vi "commander7.vi"() -> ()   [LabVIEW 2015]
uses:
  G_DATA.vi
  G_LCM.vi
  G_VEH.vi
  G_NAV.vi
  G_PATH.vi
  <vilib>/addons/control/pid/pid.llb/PID (DBL).vi
  G_SEN.vi
  <vilib>/addons/control/pid/NI_PID_pid.lvlib
panel:
  in  "handle":dbl
  in  "shifthold":dbl=0.02
  out "String":string="콜 서비스 대기 중"
  out "EURECAR_VISION":T1
  out "count":i32
  out "P2V Sign":picture[](array[picture])=[bytes[7530], bytes[7530], bytes[7530], bytes[7530]]
  out "Array 2":picture[](array[picture])
  out "sign 2":picture[](array[picture])
  out "sign":picture[](array[picture])
  in  "TTL":bool
  in  "Steering gain":dbl=0.8
  out "obs shift":dbl format="%.2f"
  in  "lane keep":bool
  in  "replay":bool
  in  "x":dbl min=-5.0 max=5.0 step=1.0
  out "display":u32=10
  out "control":u32=10
  out "update":bool=TRUE
  in  "save lcm":bool
  out "LCM Recv Data":string="GGA_2\t266\rSDT_GPS_DATA\t268\rGGA_1\t268\rRMC_2\t259\rRMC_1\t262\rEYE_RAW_T\t537\rPATH_T\t1344\rIBEO_2202_T\t672\rPOS_T\t3572\rCON_T\t4009\rCAN_T\t4707\r"
  out "GPS DATA 2":T2={"type"="WAAS", "x_lcc"=-395.2637182511565, "y_lcc"=-852.8277788987846, "latdev"=0.99, "londev"=0.99, "sats"=11, "gps_l1_ranges"=0, "gps_l1_mask_ranges"=0, "gps_l2_mask_ranges"=0, "Heading"=151.74409645131422, "lon"=127.35651, "lat"=36.36776, "time"="15:03:34.8", "hgps"=151.54, "lag"=0.0, "MAP"="KAIST"} {"lag" format="%#_5g"; "hgps" format="%#_5g"; "lat" format="%#_11g"; "lon" format="%#_11g"; "Heading" format="%#_5g"; "latdev" format="%#_4g"; "londev" format="%#_4g"}
  in  "Obs":bool=TRUE
  in  "Log":bool
  out "path":u32=10
  out "sensor":u32=10 format="%02.0f"
  out "Speed limit":dbl=20.0
  out "collision":bool
  in  "Load Path":bool
  in  "Max. Vel.":dbl=20.0 min=-5.0 max=120.0 step=5.0
  in  "RESET PATH":bool
  out "col":i16(graph)
  out "stop":bool
  in  "Reverse":bool
  in  "STOP":bool
  out "Waveform Chart 4":cluster{"auto":i16, "run":i16}(graph)={"auto"=1, "run"=0}
  out "Waveform Chart 3":cluster{"Steer_input":dbl, dbl, "handle":dbl}(graph)
  out "Waveform Chart 2":T3(graph)={"VS_des"=0.0, "VS_can"=31.498562500000002, "VS_des"=20.0}
  out "Heading":cluster{"Heading":dbl, "hgps":dbl}(graph)={"Heading"=151.74409645131422, "hgps"=151.54}
  out "XY Graph 2":cluster{"Y":dbl[], "Y":dbl[]}[](graph)=[{"Y"=[-395.3040396828474], "Y"=[-852.7527551292769]}, {"Y"=array[29298 elements], "Y"=array[29298 elements]}, {"Y"=array[29298 elements], "Y"=array[29298 elements]}, {"Y"=[-390.58210518912017], "Y"=[-861.284610912867]}]
  out "Gauge":cluster{dbl, dbl, dbl}(knob)={0.0, 31.498562500000002, 20.0} scale=-20.0..140.0
  out "Meter":cluster{dbl, dbl, dbl}(knob)={-3.5333877271700453, -5.2, -7.217874503679048} scale=-550.0..550.0
  out "XY Graph":cluster{"Y":dbl[], "Y":dbl[]}[](graph)=[{"Y"=array[11233 elements], "Y"=array[11233 elements]}, {"Y"=[-0.0, 0.0027755521495791413, 0.011103235155417224, 0.024986130588096955, 0.04442938073793812, 0.0694401981527264, 0.10002787904836907, 0.13620382065079895, 0.17798154254490584, 0.22537671212434418, 0.2784071742547809, 0.3370929852830926, 0.40145645154536425, 0.4715221725490224, 0.5473170890276435, 0.6288705360921867, 0.7162143017295008, 0.8093826909282242, 0.9084125957438758, 1.0133435716494645, 1.1242179205557647, 1.2410807809266515, 1.3639802254602955, 1.4929673668571652, 1.6280964722509026, 1.769425086939485, 1.9170141681219874, 2.0709282294217246, 2.2312354970611636, 2.3980080786478197, 2.5713221456362234], "Y"=[0.0, 0.5, 1.0, 1.5, 2.0, 2.5, 3.0, 3.5, 4.0, 4.5, 5.0, 5.5, 6.0, 6.5, 7.0, 7.5, 8.0, 8.5, 9.0, 9.5, 10.0, 10.5, 11.0, 11.5, 12.0, 12.5, 13.0, 13.5, 14.0, 14.5, 15.0]}, {"Y"=[-0.40885366553013214], "Y"=[0.1442103688222703]}, {"Y"=array[212 elements], "Y"=array[212 elements]}, {"Y"=[-0.925, -0.925, -0.925, -0.6775, -0.6775, -0.925, -0.925, -0.925, -0.925, -0.6775, -0.6775, -0.925, -0.925, -0.925, 0.9025, 0.9025, 0.9025, 0.6775, 0.6775, 0.9025, 0.9025, 0.9025, 0.9025, 0.6775, 0.6775, 0.9025, 0.9025, 0.9025, -0.925], "Y"=[-0.75, -0.224, 0.224, 0.224, -0.224, -0.224, 0.224, 2.415, 2.885, 2.885, 2.415, 2.415, 2.885, 3.5, 3.5, 2.885, 2.415, 2.415, 2.885, 2.885, 2.415, 0.224, -0.224, -0.224, 0.224, 0.224, -0.224, -0.75, -0.75]}, {"Y"=[0.0, 0.0, 0.0, 0.0, 0.0, 0.0, 0.0, 0.0, 0.0, 0.0], "Y"=[0.0, 0.5, 1.0, 1.5, 2.0, 2.5, 3.0, 3.5, 4.0, 4.5]}, {"Y"=[1.41796875, 1.3798326583616436, 1.3415997434556484, 1.3032752327956258, 1.2648643538951874, 1.226372334267944, 1.1878044014275073, 1.1491657828874886, 1.110461706161499, 1.07169739876315], "Y"=[0.0, 0.5, 1.0, 1.5, 2.0, 2.5, 3.0, 3.5, 4.0, 4.5]}, {"Y"=[-2.5234375, -2.5105986626297234, -2.4915998479127883, -2.466420726940036, -2.4350409708023073, -2.3974402505904435, -2.3535982373952864, -2.303494602307677, -2.247109016418457, -2.184421150818467], "Y"=[0.0, 0.5, 1.0, 1.5, 2.0, 2.5, 3.0, 3.5, 4.0, 4.5]}, {"Y"=[0.0, 0.0, 0.0, 0.0, 0.0, 0.0, 0.0, 0.0, 0.0, 0.0, 0.0, 0.0, 0.0, 0.0, 0.0, 0.0, 0.0, 0.0, 0.0, 0.0], "Y"=[0.0, 0.5, 1.0, 1.5, 2.0, 2.5, 3.0, 3.5, 4.0, 4.5, 5.0, 5.5, 6.0, 6.5, 7.0, 7.5, 8.0, 8.5, 9.0, 9.5]}]
  in  "Make WPT":bool
  # "e"
  # "V2I Traffic Signal"
  # "CNN\nSign\nDetection"
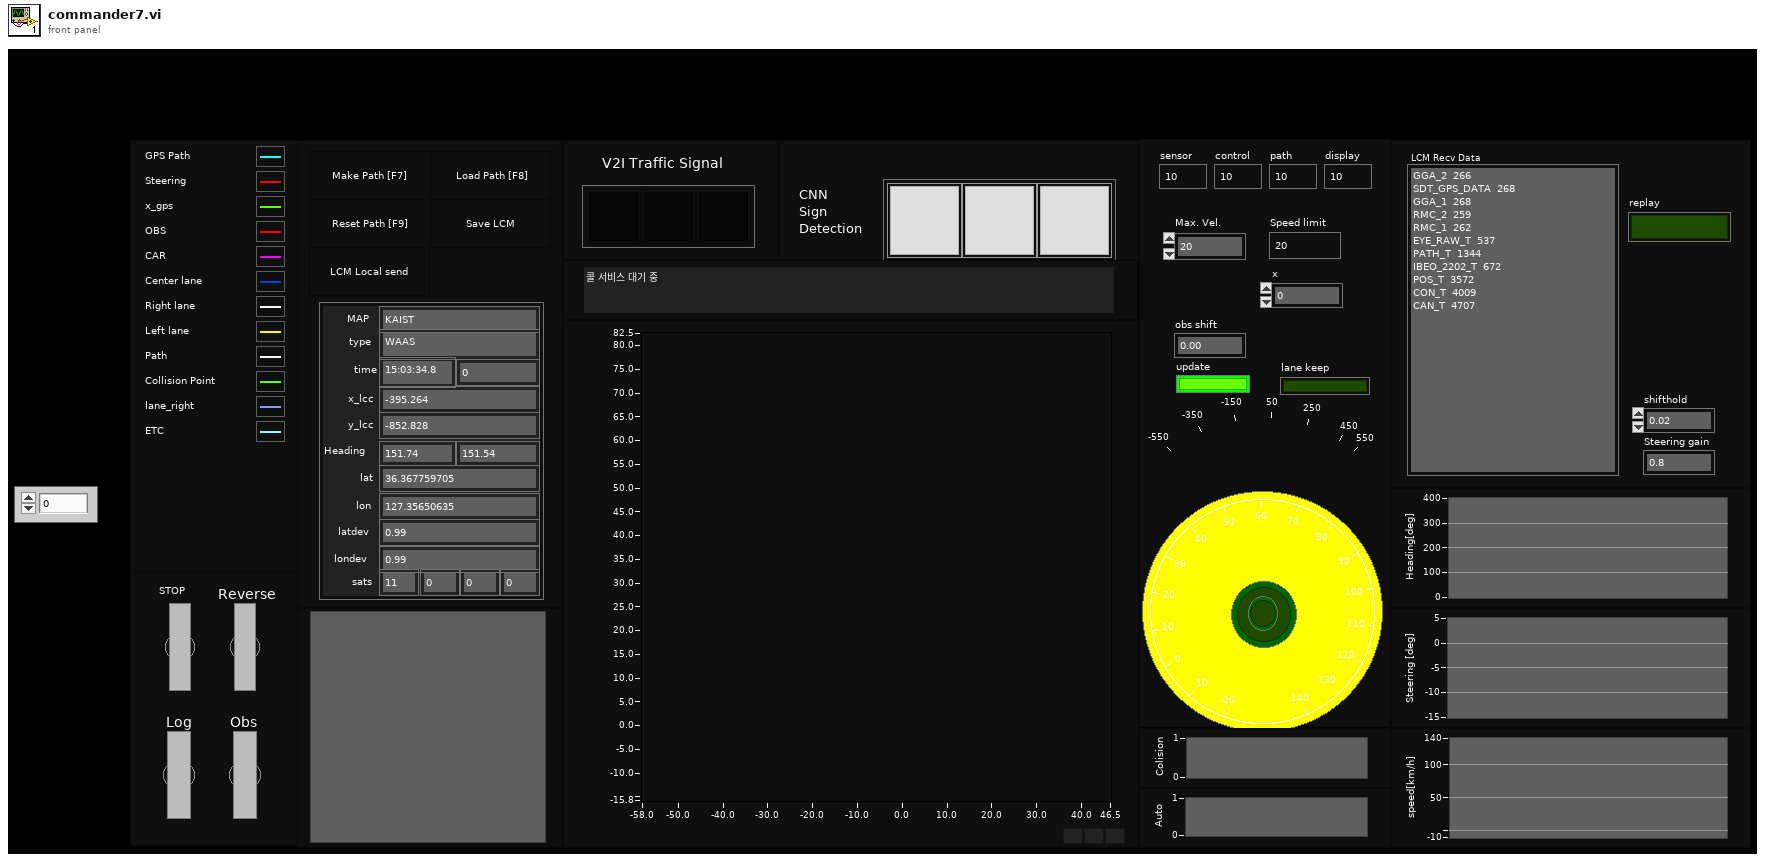
[diagram p1: front panel]
types:
  T1 = cluster{"hash":i64, "sys time":i64, "status":i32, "TS_num":i32, "TS_type":i32[], "TS_loc_x":dbl[], "TS_loc_y":dbl[]}
  T2 = cluster{"type":string, "x_lcc":dbl, "y_lcc":dbl, "latdev":sgl, "londev":sgl, "sats":u8, "gps_l1_ranges":u8, "gps_l1_mask_ranges":u8, "gps_l2_mask_ranges":u8, "Heading":dbl, "lon":sgl, "lat":sgl, "time":string, "hgps":dbl, "lag":dbl, "MAP":string}
  T3 = cluster{"VS_des":dbl, "VS_can":dbl, "VS_des":dbl}
  T4 = enum8{"Enabled", "Disabled", "Disabled and Grayed Out"}
  T5 = cluster{"proportional gain (Kc)":dbl, "integral time (Ti, min)":dbl, "derivative time (Td, min)":dbl}
  T6 = cluster{"idx":i32, "x":dbl, "y":dbl, "h":dbl, "x_path":dbl}
  T7 = cluster{"idx":i32, "x":dbl, "y":dbl, "hp":dbl, "x_path":dbl}
  T8 = cluster{"Steer_input":dbl, "Steer_output":dbl, "VS_des":dbl, "VS_can":dbl, "heading":dbl, "auto":bool, "run":bool, "x":dbl, "y":dbl}
  T9 = cluster{"X":cluster{"idx":i32, "x":dbl, "y":dbl, "h":dbl, "x_path":dbl}}[]
  T10 = typedef "imagedata.ctl" = cluster{"image type":i32, "image depth":i32, "image":u8[], "mask":u8[], "colors":u32[], "Rectangle":cluster{"left":i16, "top":i16, "right":i16, "bottom":i16}}
  T11 = cluster{"hash":i64, "sys time":i64, "s_lat":dbl, "s_lon":dbl, "d_lat":dbl, "d_lon":dbl, "Message":i64}
  T12 = cluster{"GPSTime":dbl, "attitude[2]":dbl, "lcc[0]":dbl, "lcc[1]":dbl, "heading_GPS":dbl}
  T13 = cluster{"Minimum":dbl, "Minimum":dbl, "Minimum":dbl, "Minimum":dbl, "Minimum":dbl}
  T14 = cluster{"X":cluster{"c_idx":i32, "xc":dbl, "yc":dbl, "hc":dbl, "xc_path":dbl}}[]
  T15 = cluster{"hash":i64, "sys time":i64, "time":dbl, "x":dbl, "y":dbl, "h":dbl, "numSV":i32, "postype":i32, "lag":i32, "hordev":dbl, "lat":dbl, "lon":dbl, "hgt":dbl, "map_idx":i32}
  T16 = cluster{"identifier":u32, "timestamp":timestamp, "payload":u8[]}
  T17 = cluster{"hash":i64, "sys time":i64, "size":i32, "data":u8[]}
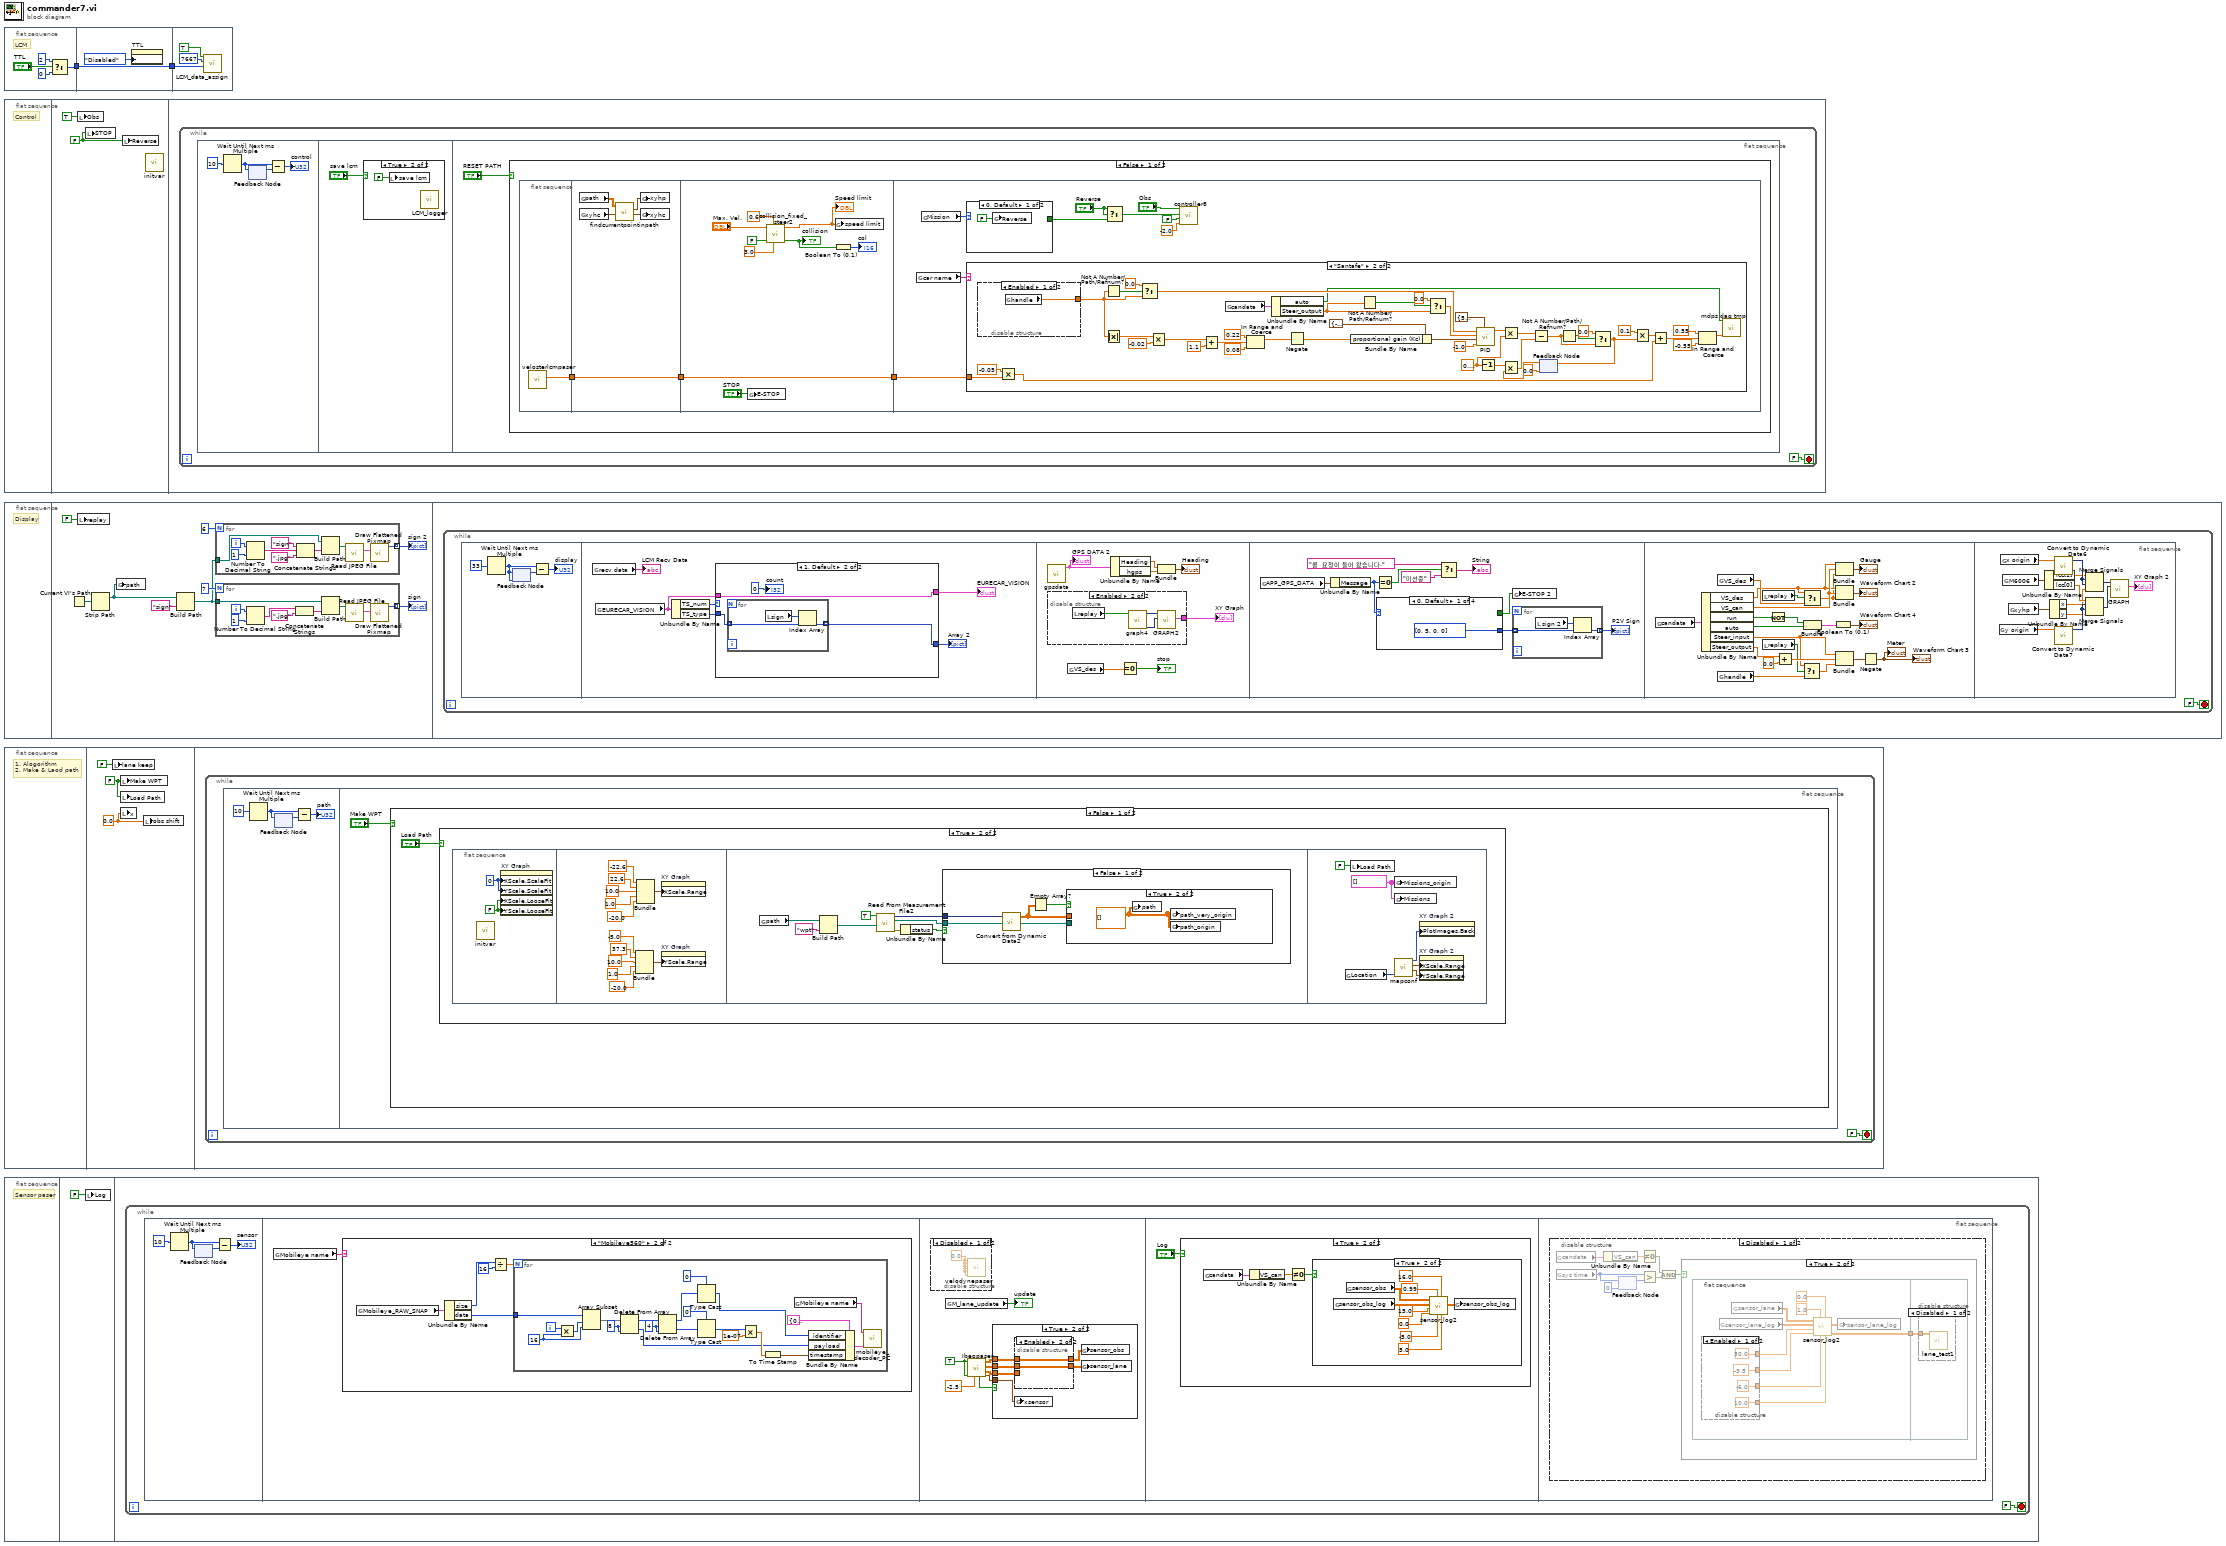
[diagram p0: block diagram]
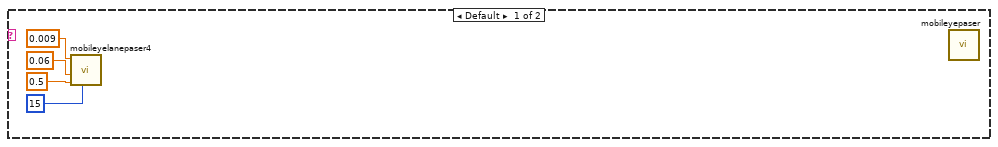
[diagram p2: hidden frame]
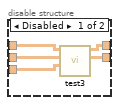
[diagram p5: hidden frame]
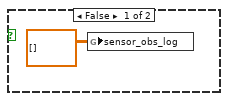
[diagram p6: hidden frame]
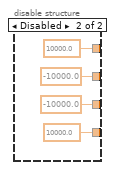
[diagram p9: hidden frame]
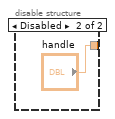
[diagram p14: hidden frame]
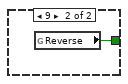
[diagram p15: hidden frame]
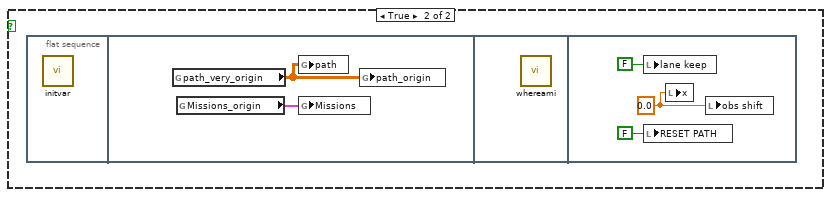
[diagram p16: hidden frame]
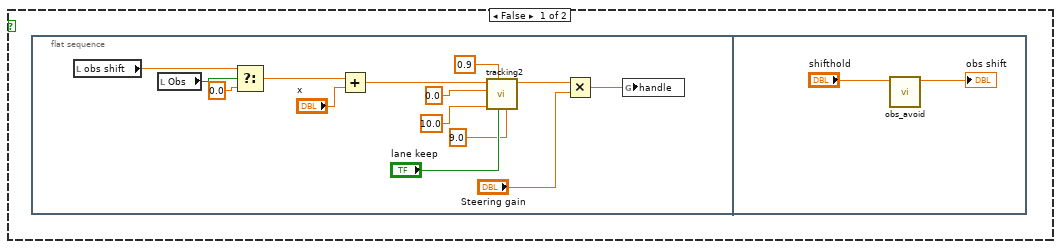
[diagram p17: hidden frame]
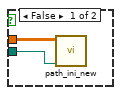
[diagram p18: hidden frame]
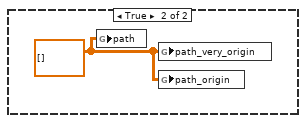
[diagram p19: hidden frame]
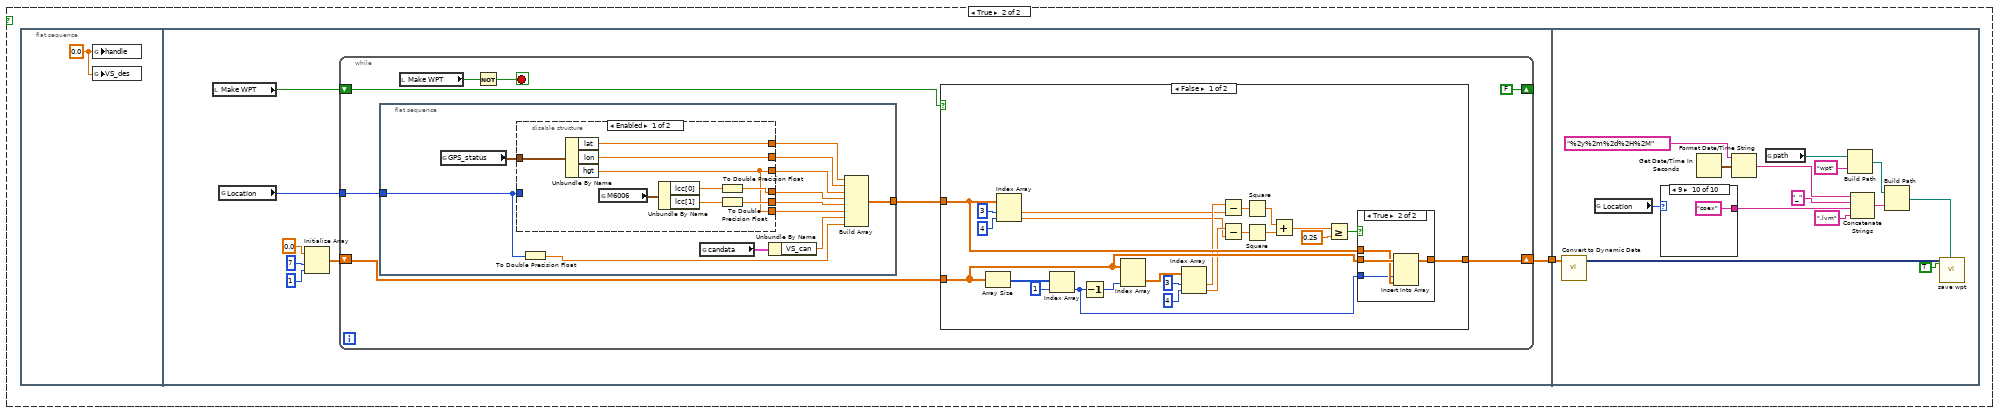
[diagram p20: hidden frame]
diagram:
  n1 = flat-sequence {
    tunnel: [w3] -> w1
    tunnel: [w8] -> w2
    tunnel: w1 -> [w8]
    tunnel: w2 -> [w11]
    frame #0 {
      # "LCM"
      n2 = Select(t=u16 2 ("time-to-live"), s="TTL", f=u16 0 ("time-to-live")) -> (s? t:f=w3:u16)
    }
    frame #1 {
      n3 = property on="TTL" class="Bool (strict)"("DisabledEnum"=T4."Disabled" ("Disabled")) -> ()  [unwired: 2 in, 2 out]
    }
    frame #2 {
      n4 = call "LCM_data_assign.vi"("time-to-live"=w11, "port"=u16 7667, "velodyne enable"=TRUE) -> ()  [unwired: 9 in]
    }
  }
  n5 = flat-sequence {
    frame #0 {
      # "Control"
    }
    frame #1 {
      w13 = FALSE ("LCM")
      n6 = local write "Obs"(TRUE ("obs")) -> ()
      n7 = local write "STOP"(w13) -> ()
      n8 = local write "Reverse"(w13) -> ()
      n9 = call "initvar.vi"() -> ()  [unwired: 12 in]
    }
    frame #2 {
      n10 = while {
        stop <- FALSE ("Loop 1") stop-if-true
        n11 = flat-sequence {
          frame #0 {
            n12 = Wait Until Next ms Multiple(millisecond multiple=u32 10 ("milliseconds to wait")) -> (millisecond timer value=w15:u32)
            n13 = feedback #1() -> (w16:u32)  [unwired: 1 in]
            n14 = feedback-in #1(w15) -> ()
            n15 = Subtract(x=w15, y=w16) -> (x-y=→"control":u32)
          }
          frame #1 {
            n16 = case shown="True" "save lcm" {
              frame False {
              }
              frame True {
                n17 = local write "save lcm"(FALSE ("save lcm")) -> ()
                n18 = call "LCM_logger.vi"() -> ()  [unwired: 12 in]
              }
            }
          }
          frame #2 {
            n19 = case shown="False" "RESET PATH" {
              frame False {
                n20 = flat-sequence {
                  tunnel: [w25] -> w24
                  tunnel: w24 -> [w26]
                  tunnel: [w26] -> w23
                  tunnel: w23 -> [w35]
                  tunnel: [w35] -> w22
                  tunnel: w22 -> [w42]
                  frame #0 {
                    n21 = call "velosterlcmpaser.vi"() -> ("mdps torque"=w25:dbl)  [unwired: 10 in, 1 out]
                  }
                  frame #1 {
                    n22 = global read "G_PATH.vi" "path"() -> (w28:dbl[][])
                    n23 = global read "G_VEH.vi" "xyhc"() -> (w29:T6)
                    n24 = call "findcurrentpointinpath.vi"("xyhc_in"=w29, "path_updated"=w28) -> ("xyhc_out"=w27:T6, "xyhp"=w30:T7)  [unwired: 8 in]
                    n25 = global write "G_VEH.vi" "xyhp"(w30) -> ()
                    n26 = global write "G_VEH.vi" "xyhc"(w27) -> ()
                  }
                  frame #2 {
                    n27 = global write "G_VEH.vi" "E-STOP"("STOP") -> ()
                    n28 = call "collision_fixed_steer2.vi"("safe  dist"=3.0, "y"=0.6 ("gaingaingain"), "obsclose"=FALSE, "Max. Vel."="Max. Vel.") -> ("collision"=w32:bool, "speed limit"=w31:dbl)  [unwired: 6 in]
                    "collision" <- w32
                    "Speed limit" <- w31
                    n29 = Boolean To (0,1)(Boolean=w32) -> (0, 1=→"col":i16)
                    n30 = global write "G_VEH.vi" "speed limit"(w31) -> ()
                  }
                  frame #3 {
                    n31 = global read "G_LCM.vi" "car name"() -> (w43:string)
                    n32 = global read "G_PATH.vi" "Mission"() -> (w48:i32)
                    n33 = case shown="0, Default" w48 {
                      tunnel: [_ w95] -> w45
                      frame 0, Default {
                        n34 = global write "G_VEH.vi" "Reverse"(FALSE ("Reverse")) -> ()
                      }
                      frame 9 {
                        n35 = global read "G_VEH.vi" "Reverse"() -> (w95:bool)
                      }
                    }
                    n36 = case shown="\"Santafe\"" w43 {
                      tunnel: w42 -> [_ w82]
                      frame "False", Default {
                      }
                      frame "Santafe" {
                        w71 = 0.6000000000000001 ("y")
                        n37 = disable-structure shown="Enabled" {
                          disable-tunnel: [w92 "handle"] -> w49
                          frame Enabled {
                            n38 = global read "G_VEH.vi" "handle"() -> (w92:dbl)
                          }
                          frame Disabled {
                          }
                        }
                        n39 = Multiply(x=-0.05 ("x 5"), y=w82) -> (x*y=w80:dbl)
                        n40 = Not A Number/Path/Refnum?(number/path/refnum=w49) -> (NaN/Path/Refnum?=w74:bool)
                        n41 = Absolute Value(x=w49) -> (abs(x)=w65:dbl)
                        n42 = Select(t=0.0, s=w74, f=w49) -> (s? t:f=w73:dbl)
                        n43 = Multiply(x=w65, y=-0.02) -> (x*y=w63:dbl)
                        n44 = Add(x=w63, y=1.1) -> (x+y=w61:dbl)
                        n45 = global read "G_VEH.vi" "candata"() -> (w91:T8)
                        n46 = In Range and Coerce(upper limit=0.22, x=w61, lower limit=0.08) -> (coerced(x)=w58:dbl)  [unwired: 1 out]
                        n47 = Unbundle By Name(w91) -> ("auto"=w50:bool, "Steer_output"=w77:dbl)
                        n48 = Negate(x=w58) -> (-x=w56:dbl)
                        n49 = Bundle By Name(cluster=T5 {"proportional gain (Kc)"=-0.1, "integral time (Ti, min)"=0.0, "derivative time (Td, min)"=0.0} ("PID gains"), "proportional gain (Kc)"=w56) -> (w55:T5)
                        n50 = Not A Number/Path/Refnum?(number/path/refnum=w77) -> (NaN/Path/Refnum?=w79:bool)
                        n51 = Select(t=0.0, s=w79, f=w77) -> (s? t:f=w76:dbl)
                        n52 = call-poly <vilib>:"PID.vi"("output range"=cluster{"output high":dbl, "output low":dbl} {"output high"=5.0, "output low"=-5.0}, "dt (s)"=-1.0, "PID gains"=w55, "process variable"=w76, "setpoint"=w73) -> ("output"=w72:dbl)  [unwired: 5 in, 1 out]
                        n53 = Decrement(x=w71) -> (x-1=w70:dbl)
                        n54 = Multiply(x=w72, y=w71) -> (x*y=w67:dbl)
                        n55 = feedback #2(0.0) -> (w69:dbl)
                        n56 = Multiply(x=w70, y=w69) -> (x*y=w68:dbl)
                        n57 = Subtract(x=w67, y=w68) -> (x-y=w52:dbl)
                        n58 = Not A Number/Path/Refnum?(number/path/refnum=w52) -> (NaN/Path/Refnum?=w54:bool)
                        n59 = Select(t=0.0, s=w54, f=w52) -> (s? t:f=w51:dbl)
                        n60 = feedback-in #2(w51) -> ()
                        n61 = Multiply(x=0.1 ("x 2"), y=w51) -> (x*y=w81:dbl)
                        n62 = Add(x=w81, y=w80) -> (x+y=w88:dbl)
                        n63 = In Range and Coerce(upper limit=0.55, x=w88, lower limit=-0.55) -> (coerced(x)=w87:dbl)  [unwired: 1 out]
                        n64 = call "mdps daq tmp.vi"("steering"=w87, "auto"=w50) -> ()  [unwired: 10 in]
                      }
                    }
                    n65 = Select(t="Reverse", s="Reverse", f=w45) -> (s? t:f=w46:bool)
                    n66 = call "controller8.vi"("Neg max speed"=-2.0, "vel"=FALSE, "reverse"=w46, "obs"="Obs") -> ()  [unwired: 8 in]
                  }
                }
              }
              frame True {
                n67 = flat-sequence {
                  frame #0 {
                    n68 = call "initvar.vi"() -> ()  [unwired: 12 in]
                  }
                  frame #1 {
                    n69 = global read "G_PATH.vi" "path_very_origin"() -> (w97:dbl[][])
                    n70 = global read "G_PATH.vi" "Missions_origin"() -> (w96:T9)
                    n71 = global write "G_PATH.vi" "path"(w97) -> ()
                    n72 = global write "G_PATH.vi" "Missions"(w96) -> ()
                    n73 = global write "G_PATH.vi" "path_origin"(w97) -> ()
                  }
                  frame #2 {
                    n74 = call "whereami.vi"() -> ()  [unwired: 12 in]
                  }
                  frame #3 {
                    w98 = 0.0 ("x")
                    n75 = local write "lane keep"(FALSE ("lane keep")) -> ()
                    n76 = local write "RESET PATH"(FALSE ("RESET PATH")) -> ()
                    n77 = local write "x"(w98) -> ()
                    n78 = local write "obs shift"(w98) -> ()
                  }
                }
              }
            }
          }
        }
      }
    }
  }
  n79 = flat-sequence {
    frame #0 {
      # "Display"
    }
    frame #1 {
      n80 = Current VI's Path() -> (path=w108:path)
      n81 = local write "replay"(FALSE ("replay")) -> ()
      n82 = Strip Path(path=w108) -> (stripped path=w101:path)  [unwired: 1 out]
      n83 = global write "G_DATA.vi" "path"(w101) -> ()
      n84 = Build Path(base path=w101, name or relative path="sign") -> (appended path=w102:path)
      n85 = for {
        N: 6 -> [_]
        tunnel: [w118] -> w104 mode=indexing
        tunnel: w102 -> [w113]
        i -> [w117]
        n86 = Number To Decimal String(number=w117, width (-)=i16 1) -> (decimal integer string=w115:string)
        n87 = Concatenate Strings("sign" ("string"), w115, ".jpg") -> (w112:string)
        n88 = Build Path(base path=w113, name or relative path=w112) -> (appended path=w111:path)
        n89 = call <vilib>:"Read JPEG File.vi"("path to JPEG file"=w111) -> ("image data"=w119:T10)  [unwired: 8 in, 2 out]
        n90 = call <vilib>:"Draw Flattened Pixmap.vi"("image data"=w119) -> ("new picture"=w118:picture)  [unwired: 8 in]
      }
      "sign 2" <- w104
      n91 = for {
        N: 7 -> [_]
        tunnel: [w127] -> w105 mode=indexing
        tunnel: w102 -> [w122]
        i -> [w126]
        n92 = Number To Decimal String(number=w126, width (-)=i16 1) -> (decimal integer string=w124:string)
        n93 = Concatenate Strings(w124, ".jpg") -> (w121:string)
        n94 = Build Path(base path=w122, name or relative path=w121) -> (appended path=w120:path)
        n95 = call <vilib>:"Read JPEG File.vi"("path to JPEG file"=w120) -> ("image data"=w128:T10)  [unwired: 8 in, 2 out]
        n96 = call <vilib>:"Draw Flattened Pixmap.vi"("image data"=w128) -> ("new picture"=w127:picture)  [unwired: 8 in]
      }
      "sign" <- w105
    }
    frame #2 {
      n97 = while {
        stop <- FALSE ("Loop 2") stop-if-true
        n98 = flat-sequence {
          frame #0 {
            n99 = Wait Until Next ms Multiple(millisecond multiple=u32 33 ("milliseconds to wait")) -> (millisecond timer value=w130:u32)
            n100 = feedback #3(w130) -> (w132:u32)
            n101 = feedback-in #3(w130) -> ()
            n102 = Subtract(x=w130, y=w132) -> (x-y=→"display":u32)
          }
          frame #1 {
            n103 = global read "G_LCM.vi" "recv data"() -> (→"LCM Recv Data":string)
            n104 = global read "G_LCM.vi" "EURECAR_VISION"() -> (w136:T1)
            n105 = Unbundle By Name(w136) -> ("TS_num"=w139:i32, "TS_type"=w138:i32[])
            n106 = case shown="1, Default" w139 {
              tunnel: w138 -> [_ w154]
              tunnel: [w147 w153] -> w137
              tunnel: w136 -> [_ w151]
              tunnel: [w140 w151] -> w135
              frame 0 {
                w149 = 100 ("x")
                n107 = local read "count"() -> (w150:i32)
                n108 = Increment(x=w150) -> (x+1=w145:i32)
                n109 = Max & Min(x=w149, y=w145) -> (min(x,y)=w144:i32)  [unwired: 1 out]
                n110 = local read "EURECAR_VISION"() -> (w141:T1)
                n111 = local write "count"(w144) -> ()
                n112 = Equal?(x=w149, y=w144) -> (x = y?=w143:bool)
                n113 = local read "Array 2"() -> (w146:picture[])
                n114 = Select(t=T1 {"hash"=0, "sys time"=0, "status"=0, "TS_num"=0, "TS_type"=[], "TS_loc_x"=[], "TS_loc_y"=[]} ("EURECAR_VISION"), s=w143, f=w141) -> (s? t:f=w140:T1)
                n115 = Select(t=picture[] [], s=w143, f=w146) -> (s? t:f=w147:picture[])
              }
              frame 1, Default {
                n116 = for {
                  tunnel: w154 -> [w156] mode=indexing
                  tunnel: [w155] -> w153 mode=indexing
                  n117 = local read "sign"() -> (w157:picture[])
                  n118 = Index Array(array=w157, index=w156) -> (element=w155:picture)
                }
                "count" <- 0 ("Numeric Control")
              }
            }
            "Array 2" <- w137
            "EURECAR_VISION" <- w135
          }
          frame #2 {
            n119 = call "gpsdata.vi"() -> ("GPS DATA 2"=w160:T2)  [unwired: 11 in]
            "GPS DATA 2" <- w160
            n120 = disable-structure shown="Enabled" {
              disable-tunnel: [w165 w170] -> w158
              frame Disabled {
                n121 = call "graph3.vi"("replay"="replay") -> ("XY Graph"=w165:cluster{"Y":dbl[], "Y":dbl[]}[])  [unwired: 9 in, 1 out]
              }
              frame Enabled {
                n122 = local read "replay"() -> (w167:bool)
                n123 = call "graph4.vi"("replay"=w167) -> ("y"=w168:dynamicdata, "x"=w169:dynamicdata)  [unwired: 9 in]
                n124 = call "GRAPH2"("Y Input"=w168, "X Input"=w169) -> ("XY Graph"=w170:cluster{"Y":dbl[], "Y":dbl[]}[])  [unwired: 3 in, 6 out]
              }
            }
            "XY Graph" <- w158
            n125 = global read "G_VEH.vi" "VS_des"() -> (w164:dbl)
            n126 = Unbundle By Name(w160) -> ("Heading"=w162:dbl, "hgps"=w161:dbl)
            n127 = Equal To 0?(x=w164) -> (x = 0?=→"stop":bool)
            n128 = Bundle("Heading"=w162, "hgps"=w161) -> (→"Heading":cluster{"Heading":dbl, "hgps":dbl})  [unwired: 1 in]
          }
          frame #3 {
            n129 = global read "G_LCM.vi" "APP_GPS_DATA"() -> (w176:T11)
            n130 = Unbundle By Name(w176) -> ("Message"=w175:i64)
            n131 = Equal To 0?(x=w175) -> (x = 0?=w174:bool)
            n132 = case shown="0, Default" w175 {
              tunnel: [_ TRUE _ _] -> w179
              tunnel: [i32[] [0, 5, 0, 0] i32[] [1, 5, 0, 0] i32[] [0, 2, 0, 0] i32[] [0, 5, 3, 0]] -> w178
              frame 0, Default {
              }
              frame 1 {
              }
              frame 2 {
              }
              frame 3 {
              }
            }
            n133 = Select(t="콜  요청이 들어 왔습니다.", s=w174, f="미션중") -> (s? t:f=→"String":string)
            n134 = global write "G_VEH.vi" "E-STOP 2"(w179) -> ()
            n135 = for {
              tunnel: w178 -> [w186] mode=indexing
              tunnel: [w185] -> w177 mode=indexing
              n136 = local read "sign 2"() -> (w187:picture[])
              n137 = Index Array(array=w187, index=w186) -> (element=w185:picture)
            }
            "P2V Sign" <- w177
          }
          frame #4 {
            n138 = global read "G_VEH.vi" "candata"() -> (w209:T8)
            n139 = Unbundle By Name(w209) -> ("VS_des"=w190:dbl, "VS_can"=w202:dbl, "run"=w200:bool, "auto"=w201:bool, "Steer_input"=w194:dbl, "Steer_output"=w199:dbl)
            n140 = global read "G_VEH.vi" "VS_des"() -> (w191:dbl)
            n141 = global read "G_VEH.vi" "handle"() -> (w195:dbl)
            n142 = local read "replay"() -> (w192:bool)
            n143 = local read "replay"() -> (w196:bool)
            n144 = Not(x=w200) -> (.not. x?=w204:bool)
            n145 = Add(x=w199, y=0.0) -> (x+y=w197:dbl)
            n146 = Select(t=w194, s=w196, f=w195) -> (s? t:f=w193:dbl)
            n147 = Select(t=w190, s=w192, f=w191) -> (s? t:f=w189:dbl)
            n148 = Bundle(w204, "auto"=w201) -> (w206:cluster{bool, "auto":bool})  [unwired: 1 in]
            n149 = Boolean To (0,1)(Boolean=w206) -> (0, 1=→"Waveform Chart 4":cluster{i16, "auto":i16})
            n150 = Bundle("VS_des"=w190, "VS_can"=w202, "VS_des"=w189) -> (→"Gauge":T3)  [unwired: 1 in]
            n151 = Bundle("VS_des"=w190, "VS_can"=w202, "VS_des"=w189) -> (→"Waveform Chart 2":T3)  [unwired: 1 in]
            n152 = Bundle("Steer_input"=w194, w197, "handle"=w193) -> (w208:cluster{"Steer_input":dbl, dbl, "handle":dbl})  [unwired: 1 in]
            n153 = Negate(x=w208) -> (-x=→"Meter" →"Waveform Chart 3":cluster{"Steer_input":dbl, dbl, "handle":dbl})
          }
          frame #5 {
            n154 = global read "G_PATH.vi" "y origin"() -> (w213:dbl[])
            n155 = global read "G_PATH.vi" "x origin"() -> (w214:dbl[])
            n156 = global read "G_NAV.vi" "M6006"() -> (w218:T12)
            n157 = global read "G_VEH.vi" "xyhp"() -> (w212:T6)
            n158 = Unbundle By Name(w218) -> ("lcc[1]"=w219:dbl, "lcc[0]"=w220:dbl)
            n159 = Unbundle By Name(w212) -> ("x"=w216:dbl, "y"=w215:dbl)
            n160 = call "Convert to Dynamic Data6"("Array"=w214) -> ("Dynamic Data Type"=w222:dynamicdata)  [unwired: 3 in]
            n161 = call "Convert to Dynamic Data7"("Array"=w213) -> ("Dynamic Data Type"=w221:dynamicdata)  [unwired: 3 in]
            n162 = Merge Signals(w219, w222, w222, w216) -> (w211:dynamicdata)
            n163 = Merge Signals(w220, w221, w221, w215) -> (w210:dynamicdata)
            n164 = call "GRAPH"("Y Input"=w210, "X Input"=w211) -> ("XY Graph"=→"XY Graph 2":cluster{"Y":dbl[], "Y":dbl[]}[])  [unwired: 3 in, 6 out]
          }
        }
      }
    }
  }
  n165 = flat-sequence {
    frame #0 {
      # "1. Alogorithm\n2. Make & Laod path"
    }
    frame #1 {
      w223 = 0.0 ("x")
      w225 = FALSE ("Make WPT")
      n166 = local write "lane keep"(FALSE ("lane update")) -> ()
      n167 = local write "Make WPT"(w225) -> ()
      n168 = local write "Load Path"(w225) -> ()
      n169 = local write "x"(w223) -> ()
      n170 = local write "obs shift"(w223) -> ()
    }
    frame #2 {
      n171 = while {
        stop <- FALSE ("Loop 3") stop-if-true
        n172 = flat-sequence {
          frame #0 {
            n173 = Wait Until Next ms Multiple(millisecond multiple=u32 10 ("milliseconds to wait")) -> (millisecond timer value=w227:u32)
            n174 = feedback #4() -> (w229:u32)  [unwired: 1 in]
            n175 = feedback-in #4(w227) -> ()
            n176 = Subtract(x=w227, y=w229) -> (x-y=→"path":u32)
          }
          frame #1 {
            n177 = case shown="False" "Make WPT" {
              frame False {
                n178 = case shown="True" "Load Path" {
                  frame False {
                    n179 = flat-sequence {
                      frame #0 {
                        n180 = local read "obs shift"() -> (w235:dbl)
                        n181 = local read "Obs"() -> (w236:bool)
                        n182 = Select(t=w235, s=w236, f=0.0) -> (s? t:f=w233:dbl)
                        n183 = Add(x=w233, y="x") -> (x+y=w246:dbl)
                        n184 = call "tracking2.vi"("x 2"=9.0, "lane keep"="lane keep", "str_gain"=0.9, "Numeric 2"=10.0, "xbody"=0.0, "xt"=w246) -> ("handle"=w243:dbl)  [unwired: 4 in, 1 out]
                        n185 = Multiply(x=w243, y="Steering gain") -> (x*y=w245:dbl)
                        n186 = global write "G_VEH.vi" "handle"(w245) -> ()
                      }
                      frame #1 {
                        n187 = call "obs_avoid.vi"("shifthold"="shifthold") -> ("obs shift"=→"obs shift":dbl)  [unwired: 10 in]
                      }
                    }
                  }
                  frame True {
                    n188 = flat-sequence {
                      frame #0 {
                        w250 = FALSE ("X Scale.Loose Fit")
                        w249 = u8 0 ("X Scale.Scale Fit")
                        n189 = call "initvar.vi"() -> ()  [unwired: 12 in]
                        n190 = property on="XY Graph" class="XYGraph (strict)"("XScale.ScaleFit"=w249, "YScale.ScaleFit"=w249, "XScale.LooseFit"=w250, "YScale.LooseFit"=w250) -> ()  [unwired: 2 in, 2 out]
                      }
                      frame #1 {
                        n191 = Bundle("Minimum"=-5.0, "Minimum"=37.3, "Minimum"=10.0, "Minimum"=1.0, "Minimum"=-20.0) -> (w255:T13)  [unwired: 1 in]
                        n192 = Bundle("Minimum"=-22.6, "Minimum"=22.6, "Minimum"=10.0, "Minimum"=1.0, "Minimum"=-20.0) -> (w262:T13)  [unwired: 1 in]
                        n193 = property on="XY Graph" class="XYGraph (strict)"("XScale.Range"=w262) -> ()  [unwired: 2 in, 2 out]
                        n194 = property on="XY Graph" class="XYGraph (strict)"("YScale.Range"=w255) -> ()  [unwired: 2 in, 2 out]
                      }
                      frame #2 {
                        n195 = global read "G_DATA.vi" "path"() -> (w266:path)
                        n196 = Build Path(base path=w266, name or relative path="wpt") -> (appended path=w264:path)
                        n197 = call "Read From Measurement File2"("Filename"=w264, "Reset"=TRUE) -> ("error out"=w268:errorcluster, "Filename Out"=w263:path, "Signals"=w270:dynamicdata)  [unwired: 4 in, 3 out]
                        n198 = Unbundle By Name(w268) -> ("status"=w267:bool)
                        n199 = case shown="False" w267 {
                          tunnel: w270 -> [w272 _]
                          tunnel: w263 -> [w271 _]
                          frame False {
                            n200 = call "Convert from Dynamic Data2"("Dynamic Data Type"=w272) -> ("Array"=w274:dbl[][])  [unwired: 3 in]
                            n201 = Empty Array?(array=w274) -> (empty?=w273:bool)
                            n202 = case shown="True" w273 {
                              tunnel: w274 -> [w276 _]
                              tunnel: w271 -> [w275 _]
                              frame False {
                                n203 = call "path_ini_new.vi"("Filename Out"=w275, "WPT"=w276) -> ()  [unwired: 10 in]
                              }
                              frame True {
                                w277 = dbl[][] [] ("path_updated")
                                n204 = global write "G_PATH.vi" "path"(w277) -> ()
                                n205 = global write "G_PATH.vi" "path_very_origin"(w277) -> ()
                                n206 = global write "G_PATH.vi" "path_origin"(w277) -> ()
                              }
                            }
                          }
                          frame True {
                            w278 = dbl[][] [] ("path_updated")
                            n207 = global write "G_PATH.vi" "path"(w278) -> ()
                            n208 = global write "G_PATH.vi" "path_very_origin"(w278) -> ()
                            n209 = global write "G_PATH.vi" "path_origin"(w278) -> ()
                          }
                        }
                      }
                      frame #3 {
                        w279 = T14 [] ("Missions_origin")
                        n210 = global read "G_VEH.vi" "Location"() -> (w280:i32)
                        n211 = local write "Load Path"(FALSE ("Load WPT")) -> ()
                        n212 = global write "G_PATH.vi" "Missions_origin"(w279) -> ()
                        n213 = global write "G_PATH.vi" "Missions"(w279) -> ()
                        n214 = call "mapconf.vi"("Location"=w280) -> ("y"=w282:cluster{dbl, dbl, "y":dbl, "y":dbl, dbl}, "x"=w283:cluster{dbl, dbl, "y":dbl, "y":dbl, dbl}, "new picture"=w284:picture)  [unwired: 8 in]
                        n215 = property on="XY Graph 2" class="XYGraph (strict)"("PlotImages.Back"=w284) -> ()  [unwired: 2 in, 2 out]
                        n216 = property on="XY Graph 2" class="XYGraph (strict)"("XScale.Range"=w283, "YScale.Range"=w282) -> ()  [unwired: 2 in, 2 out]
                      }
                    }
                  }
                }
              }
              frame True {
                n217 = flat-sequence {
                  tunnel: [w289] -> w285
                  tunnel: w285 -> [w378]
                  frame #0 {
                    w286 = 0.0
                    n218 = global write "G_VEH.vi" "handle"(w286) -> ()
                    n219 = global write "G_VEH.vi" "VS_des"(w286) -> ()
                  }
                  frame #1 {
                    n220 = local read "Make WPT"() -> (w288:bool)
                    n221 = global read "G_VEH.vi" "Location"() -> (w287:i32)
                    n222 = Initialize Array(0.0 ("element"), 7 ("dimension size"), 1 ("dimension size")) -> (w290:dbl[][])
                    n223 = while {
                      shift-right: [w295] -> w289
                      shift-left: w290 -> [w297]
                      shift-right: [FALSE] -> _
                      shift-left: w288 -> [w298]
                      tunnel: w287 -> [w294]
                      stop <- w300 stop-if-true
                      n224 = flat-sequence {
                        tunnel: [w310] -> w296
                        tunnel: w294 -> [w303]
                        frame #0 {
                          n225 = global read "G_NAV.vi" "GPS_status"() -> (w302:T15)
                          n226 = disable-structure shown="Enabled" {
                            disable-tunnel: [w321 w325] -> w313
                            disable-tunnel: [w320 w324] -> w312
                            disable-tunnel: [w314 w323] -> w311
                            disable-tunnel: w302 -> [w319 w333]
                            disable-tunnel: [w318 w332] -> w309
                            disable-tunnel: [w317 w331] -> w308
                            disable-tunnel: [w314 w330] -> w307
                            disable-tunnel: w303 -> [_ w329]
                            frame Enabled {
                              n227 = Unbundle By Name(w319) -> ("lat"=w318:dbl, "lon"=w317:dbl, "hgt"=w314:dbl)
                              n228 = global read "G_NAV.vi" "M6006"() -> (w322:T12)
                              n229 = Unbundle By Name(w322) -> ("lcc[0]"=w316:dbl, "lcc[1]"=w315:dbl)
                              n230 = To Double Precision Float(number=w316) -> (double precision float=w321:dbl)
                              n231 = To Double Precision Float(number=w315) -> (double precision float=w320:dbl)
                            }
                            frame Disabled {
                              n232 = Unbundle By Name(w333) -> ("lat"=w332:dbl, "lon"=w331:dbl, "hgt"=w330:dbl)
                              n233 = call "getecefdcmref.vi"("map"=w329) -> ("XYZ"=w328:dbl[])  [unwired: 10 in, 4 out]
                              n234 = call "llh2lcc.vi"("ecef ref"=w328, "hgt"=w330, "lon"=w331, "lat"=w332) -> ("lcc"=w327:dbl[])  [unwired: 7 in]
                              n235 = Index Array(array=w327, index #1=0 ("index")) -> (element #1=w325:dbl, element #2=w324:dbl, element #3=w323:dbl)  [unwired: 2 in]
                            }
                          }
                          n236 = To Double Precision Float(number=w303) -> (double precision float=w304:dbl)
                          n237 = global read "G_VEH.vi" "candata"() -> (w306:T8)
                          n238 = Unbundle By Name(w306) -> ("VS_can"=w305:dbl)
                          n239 = Build Array(w309, w308, w307, w313, w312, w311, w305, w304) -> (w310:dbl[])
                        }
                      }
                      n240 = local read "Make WPT"() -> (w301:bool)
                      n241 = Not(x=w301) -> (.not. x?=w300:bool)
                      n242 = case shown="False" w298 {
                        tunnel: w297 -> [w348 w365]
                        tunnel: w296 -> [w347 w363]
                        tunnel: [w346 w362] -> w295
                        frame False {
                          n243 = Array Size(array=w348) -> (size(s)=w356:i32[])
                          n244 = Index Array(array=w347, index #1=3 ("index"), index #2=4 ("index")) -> (element #1=w342:dbl, element #2=w340:dbl)
                          n245 = Index Array(array=w356, index=1) -> (element=w345:i32)
                          n246 = Decrement(x=w345) -> (x-1=w344:i32)
                          n247 = Index Array(array=w348, index (col)=w344) -> (element=w352:dbl[])  [unwired: 1 in]
                          n248 = Index Array(array=w352, index #1=3 ("index"), index #2=4 ("index")) -> (element #1=w343:dbl, element #2=w341:dbl)
                          n249 = Subtract(x=w343, y=w342) -> (x-y=w339:dbl)
                          n250 = Subtract(x=w341, y=w340) -> (x-y=w338:dbl)
                          n251 = Square(x=w339) -> (x^2=w337:dbl)
                          n252 = Square(x=w338) -> (x^2=w336:dbl)
                          n253 = Add(x=w337, y=w336) -> (x+y=w335:dbl)
                          n254 = Greater Or Equal?(x=w335, y=0.25) -> (x >= y?=w349:bool)
                          n255 = case shown="True" w349 {
                            tunnel: w348 -> [w357 w361]
                            tunnel: w345 -> [_ w358]
                            tunnel: w347 -> [_ w360]
                            tunnel: [w357 w359] -> w346
                            frame False {
                            }
                            frame True {
                              n256 = Insert Into Array(array=w361, index (col)=w358, new element=w360) -> (w359:dbl[][])  [unwired: 1 in]
                            }
                          }
                        }
                        frame True {
                          n257 = Replace Array Subset(array=w365, new element=w363, index (col)=0 ("disabled index (col)")) -> (w362:dbl[][])  [unwired: 1 in]
                        }
                      }
                    }
                  }
                  frame #2 {
                    n258 = call "Convert to Dynamic Data"("2D Array"=w378) -> ("Dynamic Data Type"=w379:dynamicdata)  [unwired: 3 in]
                    n259 = global read "G_VEH.vi" "Location"() -> (w375:i32)
                    n260 = case shown="9" w375 {
                      tunnel: ["" ("String") "Hyundai" ("String") "KAIST" ("String") "AJOU" ("String") "MUNJI" ("String") "Airforce" ("String") "CAR" ("String") "KATRI" ("String") _ "coex" ("String")] -> w374
                      frame 0, Default {
                      }
                      frame 1 {
                      }
                      frame 2 {
                      }
                      frame 3 {
                      }
                      frame 4 {
                      }
                      frame 5 {
                      }
                      frame 6 {
                      }
                      frame 7 {
                      }
                      frame 8 {
                      }
                      frame 9 {
                      }
                    }
                    n261 = Get Date/Time In Seconds() -> (seconds since 1Jan1904=w376:timestamp)
                    n262 = Format Date/Time String(time format string (%c)="%2y%2m%2d%2H%2M", seconds (now)=w376) -> (date/time string=w372:string)  [unwired: 1 in]
                    n263 = global read "G_DATA.vi" "path"() -> (w370:path)
                    n264 = Build Path(base path=w370, name or relative path="wpt") -> (appended path=w368:path)
                    n265 = Concatenate Strings(w372, "_" ("string"), w374, ".lvm" ("string")) -> (w367:string)
                    n266 = Build Path(base path=w368, name or relative path=w367) -> (appended path=w366:path)
                    n267 = call "save wpt"("Signals"=w379, "Reset"=TRUE, "Filename"=w366) -> ()  [unwired: 14 in, 3 out]
                  }
                }
              }
            }
          }
        }
      }
    }
  }
  n268 = flat-sequence {
    frame #0 {
      # "Sensor paser"
    }
    frame #1 {
      n269 = local write "Log"(FALSE ("obs")) -> ()
    }
    frame #2 {
      n270 = while {
        stop <- FALSE ("Loop 4") stop-if-true
        n271 = flat-sequence {
          frame #0 {
            n272 = Wait Until Next ms Multiple(millisecond multiple=u32 10 ("milliseconds to wait")) -> (millisecond timer value=w392:u32)
            n273 = feedback #5() -> (w394:u32)  [unwired: 1 in]
            n274 = feedback-in #5(w392) -> ()
            n275 = Subtract(x=w392, y=w394) -> (x-y=→"sensor":u32)
          }
          frame #1 {
            n276 = global read "G_LCM.vi" "Mobileye name"() -> (w396:string)
            n277 = case shown="\"Mobileye560\"" w396 {
              frame Default {
                n278 = call "mobileyelanepaser4.vi"("count hold"=u64 15, "thresh  c"=0.5, "thresh  b"=0.06 ("thresh 2"), "thresh r"=0.009 ("y")) -> ()  [unwired: 4 in, 4 out]
                n279 = call "mobileyepaser.vi"() -> ()  [unwired: 11 in, 1 out]
              }
              frame "Mobileye560" {
                n280 = global read "G_LCM.vi" "Mobileye_RAW_SNAP"() -> (w401:T17)
                n281 = Unbundle By Name(w401) -> ("size"=w402:i32, "data"=w405:u8[])
                n282 = Divide(x=w402, y=16) -> (x/y=w404:dbl)
                n283 = for {
                  N: w404 -> [_]
                  tunnel: w405 -> [w425]
                  i -> [w424]
                  w417 = 4 ("length")
                  w415 = 8 ("index")
                  w423 = 16 ("y")
                  n284 = Multiply(x=w424, y=w423) -> (x*y=w422:i32)
                  n285 = Array Subset(array=w425, index=w422, length=w423) -> (w407:u8[])
                  n286 = Delete From Array(array=w407, length=w415, index=w415) -> (deleted portion=w408:u8[], array with subset deleted=w416:u8[])
                  n287 = Delete From Array(array=w416, length=w417, index=w417) -> (deleted portion=w421:u8[], array with subset deleted=w418:u8[])
                  n288 = Type Cast(type=u32 0, x=w418) -> (*(type *) &x=w409:u32)
                  n289 = Type Cast(type=u32 0, x=w421) -> (*(type *) &x=w410:u32)
                  n290 = Multiply(x=w410, y=1e-07) -> (x*y=w413:dbl)
                  n291 = To Time Stamp(1:w413) -> (0:w412:timestamp)
                  n292 = global read "G_LCM.vi" "Mobileye name"() -> (w426:string)
                  n293 = Bundle By Name(cluster=T16 {"identifier"=0, "timestamp"=timestamp(0 s since 1904-01-01), "payload"=[]} ("can cluster"), "identifier"=w409, "payload"=w408, "timestamp"=w412) -> (w406:T16)
                  n294 = call "mobileye_decoder_PC.vi"("can cluster"=w406, "name"=w426) -> ()  [unwired: 10 in]
                }
              }
            }
          }
          frame #2 {
            w429 = TRUE ("Sensor [F12]")
            n295 = disable-structure shown="Disabled" {
              frame Disabled {
                w435 = 0.0 ("roll")
                n296 = call "velodynepaser.vi"("roll"=w435, "pitch"=w435, "heading"=w435, "dX"=w435, "dY"=w435, "dZ"=w435) -> ()  [unwired: 12 in, 2 out]
              }
              frame Enabled {
              }
            }
            n297 = global read "G_SEN.vi" "M_lane_update"() -> (→"update":bool)
            n298 = call "Ibeopaser.vi"("theta"=-2.5, "Hide Transparent"=w429, "Sensor [F12]"=w429) -> ("x_sensor"=w433:T6, "etc"=w431:dbl[][], "lane"=w432:dbl[][], "obs"=w434:dbl[][], "update"=w430:bool)  [unwired: 4 in]
            n299 = case shown="True" w430 {
              tunnel: w434 -> [_ w440]
              tunnel: w433 -> [_ w441]
              tunnel: w432 -> [_ w437]
              tunnel: w431 -> [_ w438]
              frame False {
              }
              frame True {
                n300 = disable-structure shown="Enabled" {
                  disable-tunnel: w440 -> [w446 w448]
                  disable-tunnel: [w445 w448] -> w439
                  disable-tunnel: w438 -> [w444 _]
                  disable-tunnel: w437 -> [w443 w447]
                  disable-tunnel: [w442 w447] -> w436
                  frame Disabled {
                    n301 = call "test3.vi"("sensor_all"=w444, "sensor_lane"=w443, "sensor_obs"=w446) -> ("lane"=w442:dbl[][], "obs"=w445:dbl[][])  [unwired: 6 in, 1 out]
                  }
                  frame Enabled {
                  }
                }
                n302 = global write "G_VEH.vi" "xsensor"(w441) -> ()
                n303 = global write "G_SEN.vi" "sensor_obs"(w439) -> ()
                n304 = global write "G_SEN.vi" "sensor_lane"(w436) -> ()
              }
            }
          }
          frame #3 {
            n305 = case shown="True" "Log" {
              frame False {
                n306 = global write "G_SEN.vi" "sensor_obs_log"(dbl[][] [] ("sensor_obs_log")) -> ()
              }
              frame True {
                n307 = global read "G_VEH.vi" "candata"() -> (w452:T8)
                n308 = Unbundle By Name(w452) -> ("VS_can"=w453:dbl)
                n309 = Not Equal To 0?(x=w453) -> (x != 0?=w451:bool)
                n310 = case shown="True" w451 {
                  frame False {
                  }
                  frame True {
                    n311 = global read "G_SEN.vi" "sensor_obs_log"() -> (w455:dbl[][])
                    n312 = global read "G_SEN.vi" "sensor_obs"() -> (w456:dbl[][])
                    n313 = call "sensor_log2.vi"("xmax"=5.0, "range^2"=16.0, "xmin"=-5.0, "FF"=0.99 ("t"), "ymin"=0.0, "ymax"=15.0, "sensor_log"=w455, "sensor_obs"=w456) -> ("sensor_log 2"=w454:dbl[][])  [unwired: 2 in, 1 out]
                    n314 = global write "G_SEN.vi" "sensor_obs_log"(w454) -> ()
                  }
                }
              }
            }
          }
          frame #4 {
            n315 = disable-structure shown="Disabled" {
              frame Disabled {
                n316 = global read "G_VEH.vi" "candata"() -> (w469:T8)
                n317 = global read "G_VEH.vi" "sys time"() -> (w464:i64)
                n318 = Unbundle By Name(w469) -> ("VS_can"=w470:dbl)
                n319 = feedback-in #6(w464) -> ()
                n320 = feedback #6(i64 0 ("sys time")) -> (w468:i64)
                n321 = Not Equal To 0?(x=w470) -> (x != 0?=w466:bool)
                n322 = Greater?(x=w464, y=w468) -> (0:w467:bool)
                n323 = And(x=w466, y=w467) -> (x .and. y?=w465:bool)
                n324 = case shown="True" w465 {
                  frame False {
                  }
                  frame True {
                    n325 = flat-sequence {
                      tunnel: [w472] -> w471
                      tunnel: w471 -> [w490]
                      frame #0 {
                        n326 = disable-structure shown="Enabled" {
                          disable-tunnel: [50.0 ("ymax") 10000.0 ("ymax")] -> w477
                          disable-tunnel: [-3.5 ("ymin") -10000.0 ("ymin")] -> w476
                          disable-tunnel: [-6.0 ("xmin") -10000.0 ("xmin")] -> w475
                          disable-tunnel: [10.0 ("xmin") 10000.0 ("xmax")] -> w474
                          frame Enabled {
                          }
                          frame Disabled {
                          }
                        }
                        n327 = global read "G_SEN.vi" "sensor_lane_log"() -> (w481:dbl[][])
                        n328 = global read "G_SEN.vi" "sensor_lane"() -> (w480:dbl[][])
                        n329 = call "sensor_log2.vi"("xmax"=w474, "range^2"=0.0, "xmin"=w475, "FF"=1.0, "ymin"=w476, "ymax"=w477, "sensor_log"=w481, "sensor_obs"=w480) -> ("sensor_log_body"=w472:dbl[][], "sensor_log 2"=w473:dbl[][])  [unwired: 2 in]
                        n330 = global write "G_SEN.vi" "sensor_lane_log"(w473) -> ()
                      }
                      frame #1 {
                        n331 = disable-structure shown="Disabled" {
                          disable-tunnel: w490 -> [w491 _]
                          frame Disabled {
                            n332 = call "lane_test1.vi"("lane_body"=w491) -> ()  [unwired: 11 in]
                          }
                          frame Enabled {
                          }
                        }
                      }
                    }
                  }
                }
              }
              frame Enabled {
              }
            }
          }
        }
      }
    }
  }
